vi "Start Logger.vi"(8 "error in (no error)":errorcluster, 11 "Measure Controller in":refnum<class "Process Controller.lvclass">) -> (0 "error out":errorcluster, 2 "File Path":path, 3 "Measure Controller out":refnum<class "Process Controller.lvclass">)   [LabVIEW 2018, in "Process Controller.lvclass"]
uses:
  Process Controller.lvclass
  Process Controller.lvclass/Process Controller.ctl
  Read Log Init Response.vi
  Sequence Elements/Sequence Element/Sequence Element.lvclass
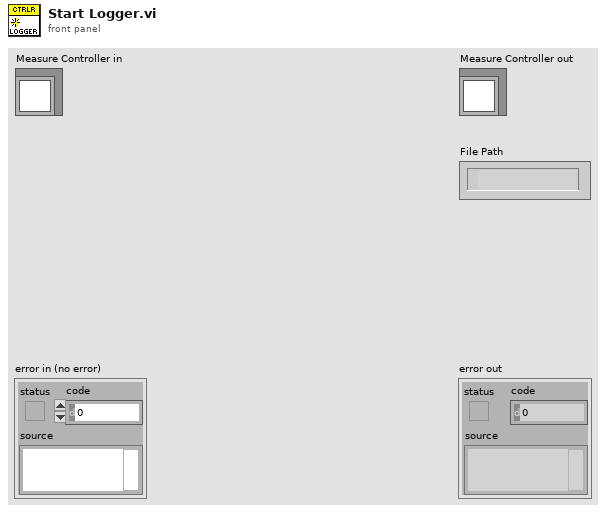
[diagram p1: front panel]
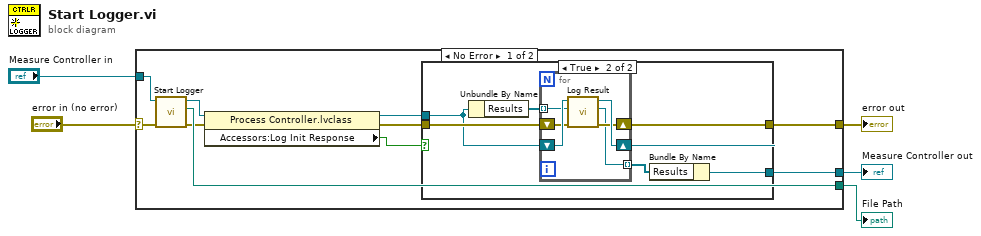
[diagram p0: block diagram]
diagram:
  n1 = case shown="No Error" "error in (no error)" {
    selector: "error in (no error)" -> [w12 w32]
    tunnel: [w13 w32] -> w4
    tunnel: [w14 w31] -> w2
    tunnel: "Measure Controller in" -> [w15 w31]
    tunnel: [w11 _] -> w1
    frame No Error {
      n2 = call-parent "Start Logger.vi"("error in (no error)"=w12, "Worker in"=w15) -> ("error out"=w10:errorcluster, "File Path"=w11:path, "Worker out"=w8:refnum<class "Process Controller.lvclass">)  [unwired: 7 in]
      n3 = property class="Process Controller.lvclass"(reference=w8, error in=w10) -> (reference out=w7:refnum<class "Process Controller.lvclass">, error out=w9:errorcluster, "Accessors:Log Init Response"=w6:bool)
      n4 = case shown="True" w6 {
        tunnel: [w16 w24] -> w14
        tunnel: [w17 w22] -> w13
        tunnel: w9 -> [w17 w19]
        tunnel: w7 -> [w16 w18]
        frame False {
        }
        frame True {
          n5 = Unbundle By Name(w18) -> ("Results"=w21:refnum<class "Acquired Result.lvclass">[])
          n6 = for {
            tunnel: w21 -> [w28] mode=indexing
            shift-right: [w26] -> w22
            shift-left: w19 -> [w27]
            tunnel: [w25] -> w23 mode=indexing
            shift-right: [w29] -> w20
            shift-left: w18 -> [w30]
            n7 = call-dynamic "Log Result.vi"("error in (no error)"=w27, "Result"=w28, "Process Controller in"=w30) -> ("error out"=w26:errorcluster, "Result out"=w25:refnum<class "Acquired Result.lvclass">, "Process Controller out"=w29:refnum<class "Process Controller.lvclass">)  [unwired: 6 in]
          }
          n8 = Bundle By Name(cluster=w20, "Results"=w23) -> (w24:refnum<class "Process Controller.lvclass">)
        }
      }
    }
    frame Error {
    }
  }
  "error out" <- w4
  "Measure Controller out" <- w2
  "File Path" <- w1
